vi "Load Settings from XML.vi"(8 "error in (no error)":errorcluster, 11 "Settings in":T1) -> (0 "error out":errorcluster, 3 "Settings out":T1)   [LabVIEW 2020, in "UI.lvlib"]
doc: "Attempts to load previous user specified settings from an XML file.\n\nThis VI will not generate an error. If a suitable XML file can't be loaded and parsed then it will simply return the default settings."
uses:
  UI.lvlib
  Settings.ctl
  Acquisition/_support/Hardware Configuration.ctl
  Acquisition/_support/Signal Type.ctl
  Logging/_support/Logging Configuration.ctl
  <vilib>/Utility/xml.llb/Read From XML File(string).vi
  <vilib>/Utility/xml.llb/Write to XML File(string).vi
  Acquisition/Acquisition.lvlib
  Logging/Logging.lvlib
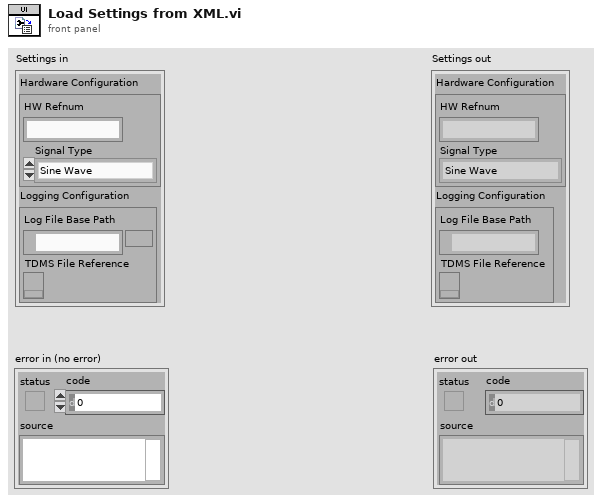
[diagram p1: front panel]
types:
  T1 = typedef "UI.lvlib/Settings.ctl" = cluster{"Hardware Configuration":T2, "Logging Configuration":T4}
  T2 = typedef "Acquisition.lvlib/Hardware Configuration.ctl" = cluster{"HW Refnum":string, "Signal Type":T3}
  T3 = typedef "Acquisition.lvlib/Signal Type.ctl" = enum16{"Sine Wave", "Square with Noise"}
  T4 = typedef "Logging.lvlib/Logging Configuration.ctl" = cluster{"Log File Base Path":path, "TDMS File Reference":refnum<k34>}
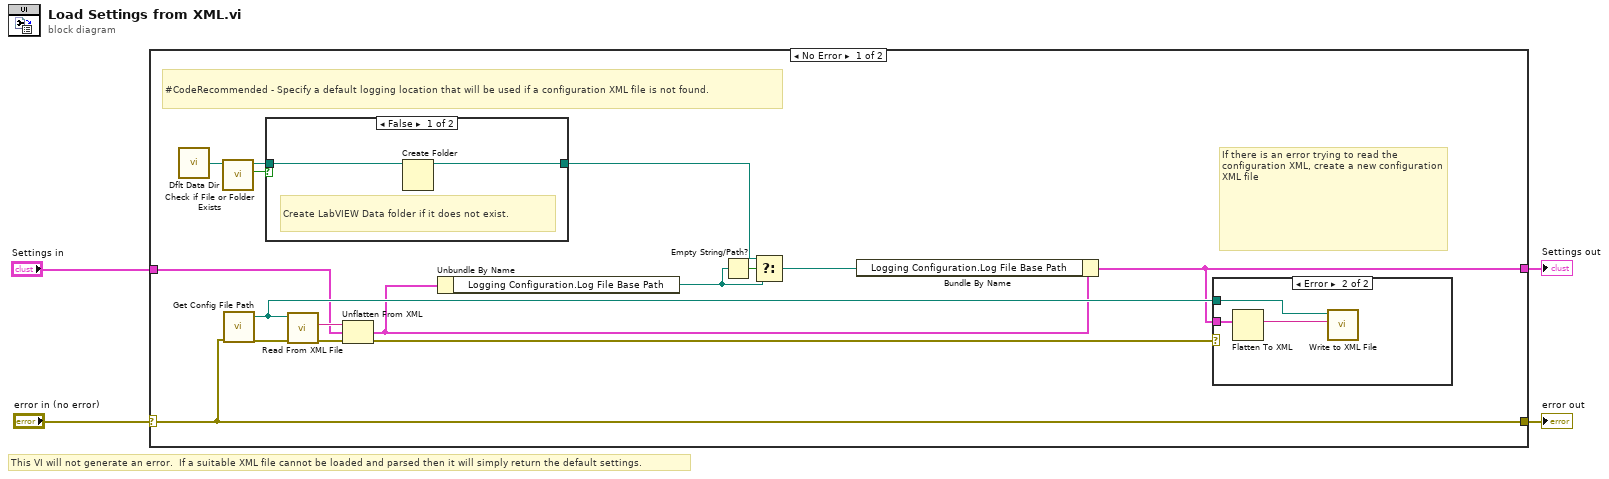
[diagram p0: block diagram]
diagram:
  # "This VI will not generate an error.  If a suitable XML file cannot be loaded and parsed then it will simply return the default settings."
  n1 = case shown="No Error" "error in (no error)" {
    selector: "error in (no error)" -> [w18 w28]
    tunnel: [w18 w28] -> w3
    tunnel: "Settings in" -> [w14 w27]
    tunnel: [w9 w27] -> w1
    frame No Error {
      # "If there is an error trying to read the configuration XML, create a new configuration XML file"
      # "#CodeRecommended - Specify a default logging location that will be used if a configuration XML file is not found."
      n2 = call <vilib>:"Dflt Data Dir.vi"() -> ("App:Default Data Directory"=w8:path)
      n3 = call <vilib>:"Check if File or Folder Exists.vi"("path"=w8) -> ("file or folder exists?"=w7:bool, "dup path"=w6:path)  [unwired: 8 in, 1 out]
      n4 = call "Get Config File Path.vi"("error in (no error)"=w18) -> ("error out"=w20:errorcluster, "XML File Path"=w17:path)  [unwired: 9 in]
      n5 = case shown="False" w7 {
        tunnel: w6 -> [w22 w23]
        tunnel: [w21 w23] -> w5
        frame False {
          # "Create LabVIEW Data folder if it does not exist."
          n6 = Create Folder(path (use dialog)=w22) -> (created path=w21:path)  [unwired: 2 in, 2 out]
        }
        frame True {
        }
      }
      n7 = call-poly <vilib>:"Read From XML File.vi"("error in (no error)"=w20, "XML File Path"=w17) -> ("error out"=w16:errorcluster, "XML Elements"=w19:string)  [unwired: 7 in, 1 out]
      n8 = Unflatten From XML(xml string=w19, type=w14, error in (no error)=w16) -> (value=w11:T1, error out=w15:errorcluster)
      n9 = Unbundle By Name(w11) -> ("Logging Configuration.Log File Base Path"=w12:path)
      n10 = Empty String/Path?(string/path=w12) -> (empty?=w13:bool)
      n11 = Select(t=w5, s=w13, f=w12) -> (s? t:f=w10:path)
      n12 = Bundle By Name(cluster=w11, "Logging Configuration.Log File Base Path"=w10) -> (w9:T1)
      n13 = case shown="Error" w15 {
        tunnel: w9 -> [_ w26]
        tunnel: w17 -> [_ w24]
        frame No Error {
        }
        frame Error {
          n14 = Flatten To XML(6:w26) -> (2:w25:string)
          n15 = call-poly <vilib>:"Write to XML File.vi"("XML Input"=w25, "XML File Path"=w24) -> ()  [unwired: 7 in, 3 out]
        }
      }
    }
    frame Error {
    }
  }
  "error out" <- w3
  "Settings out" <- w1
